vi "Hour Differences.vi"(2 "Report Data In":string[][](array[string])=[["In", "4/24/2017 9:33:33 AM", ""], ["Break", "4/24/2017 10:59:30 AM", "DoIT"], ["In", "4/24/2017 11:10:28 AM", ""], ["Out", "4/24/2017 5:24:46 PM", ""], ["In", "4/25/2017 1:06:32 PM", ""], ["Out", "4/25/2017 6:08:20 PM", ""], ["In", "4/26/2017 9:58:55 AM", ""], ["Out", "4/26/2017 4:19:40 PM", ""], ["In", "4/27/2017 9:45:36 AM", ""], ["Out", "4/27/2017 5:44:32 PM", ""], ["In", "4/28/2017 9:22:47 AM", ""], ["Break", "4/28/2017 11:17:53 AM", "Test"], ["In", "4/28/2017 11:20:31 AM", "Testing"], ["Out", "4/28/2017 11:22:16 AM", ""], ["In", "4/28/2017 11:38:38 AM", ""], ["In", "4/28/2017 11:43:36 AM", ""], ["In", "4/28/2017 11:46:33 AM", ""], ["In", "4/28/2017 11:47:05 AM", ""], ["Break", "4/28/2017 11:47:20 AM", "TESTING"], ["In", "4/28/2017 11:47:27 AM", ""]]) -> (0 "Report Data Out":string[][](array[string])=[["In", "4/24/2017 9:33:33 AM", ""], ["Break", "4/24/2017 10:59:30 AM", "DoIT"], ["In", "4/24/2017 11:10:28 AM", ""], ["Out", "4/24/2017 5:24:46 PM", ""], ["In", "4/25/2017 1:06:32 PM", ""], ["Out", "4/25/2017 6:08:20 PM", ""], ["In", "4/26/2017 9:58:55 AM", ""], ["Out", "4/26/2017 4:19:40 PM", ""], ["In", "4/27/2017 9:45:36 AM", ""], ["Out", "4/27/2017 5:44:32 PM", ""], ["In", "4/28/2017 9:22:47 AM", ""], ["Break", "4/28/2017 11:17:53 AM", "Test"], ["In", "4/28/2017 11:20:31 AM", "Testing"], ["Out", "4/28/2017 11:22:16 AM", ""], ["In", "4/28/2017 11:38:38 AM", ""], ["In", "4/28/2017 11:43:36 AM", ""], ["In", "4/28/2017 11:46:33 AM", ""], ["In", "4/28/2017 11:47:05 AM", ""], ["Break", "4/28/2017 11:47:20 AM", "TESTING"], ["In", "4/28/2017 11:47:27 AM", ""]], 1 "Total Hours":string)   [LabVIEW 2020]
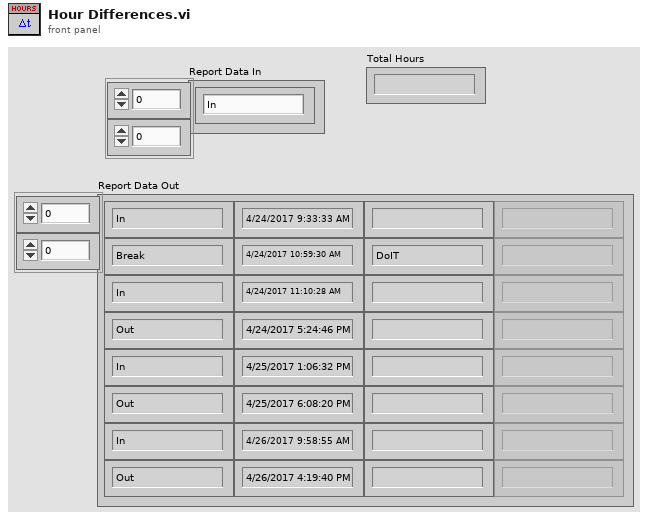
[diagram p1: front panel]
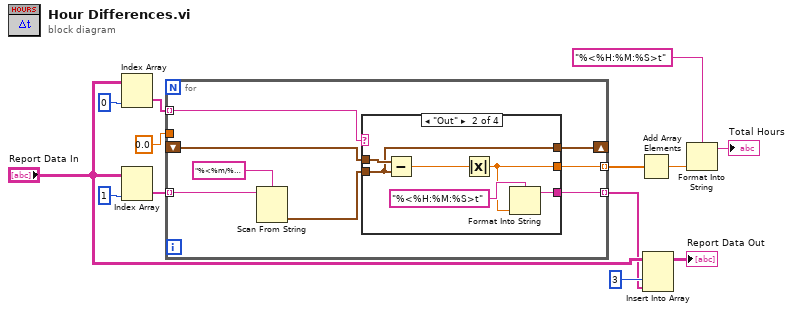
[diagram p0: block diagram]
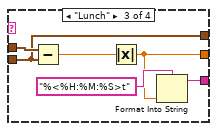
[diagram p3: hidden frame]
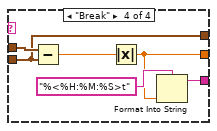
[diagram p4: hidden frame]
diagram:
  n1 = Index Array(array="Report Data In", index (col)=0 ("disabled index (col)")) -> (element=w10:string[])  [unwired: 1 in]
  n2 = Index Array(array="Report Data In", index (col)=1 ("disabled index (col)")) -> (element=w12:string[])  [unwired: 1 in]
  n3 = for {
    tunnel: w12 -> [w20] mode=indexing
    tunnel: w10 -> [w19] mode=indexing
    shift-right: [w17] -> _
    shift-left: _ -> [w16]
    tunnel: [w15] -> w7 mode=indexing
    tunnel: 0.0 -> [_]
    tunnel: [w14] -> w4 mode=indexing
    n4 = Scan From String "Scan From String"(format string="%<%m/%d/%Y %I:%M:%S%3u %p>T", input string=w20) -> (output 1=w18:timestamp)  [unwired: 3 in, 3 out]
    n5 = case shown="\"Out\"" w19 {
      tunnel: w18 -> [w22 w26 w32 w38]
      tunnel: [w22 w26 w32 w38] -> w17
      tunnel: w16 -> [_ w28 w33 w39]
      tunnel: [_ w24 w30 w36] -> w15
      tunnel: [_ w23 w29 w35] -> w14
      frame "In", Default {
      }
      frame "Out" {
        n6 = Subtract(x=w28, y=w26) -> (x-y=w27:dbl)
        n7 = Absolute Value(x=w27) -> (abs(x)=w23:dbl)
        n8 = Format Into String(format string="%<%H:%M:%S>t", w23) -> (resulting string=w24:string)  [unwired: 2 in, 1 out]
      }
      frame "Lunch" {
        n9 = Subtract(x=w33, y=w32) -> (x-y=w34:dbl)
        n10 = Absolute Value(x=w34) -> (abs(x)=w29:dbl)
        n11 = Format Into String(format string="%<%H:%M:%S>t", w29) -> (resulting string=w30:string)  [unwired: 2 in, 1 out]
      }
      frame "Break" {
        n12 = Subtract(x=w39, y=w38) -> (x-y=w40:dbl)
        n13 = Absolute Value(x=w40) -> (abs(x)=w35:dbl)
        n14 = Format Into String(format string="%<%H:%M:%S>t", w35) -> (resulting string=w36:string)  [unwired: 2 in, 1 out]
      }
    }
  }
  n15 = Add Array Elements(numeric array=w4) -> (sum=w3:dbl)
  n16 = Insert Into Array(array="Report Data In", index (col)=3 ("disabled index (col)"), new element=w7) -> (→"Report Data Out":string[][])  [unwired: 1 in]
  n17 = Format Into String(format string="%<%H:%M:%S>t", w3) -> (resulting string=→"Total Hours":string)  [unwired: 2 in, 1 out]
